vi "mass.vi"(1 "mass":dbl=1.0) -> (0 "urdf":string="<material>\n  <ambient> 0.705882 0.247059 0.000000 1.000000</ambient>\n</material>\n")   [LabVIEW 2012]
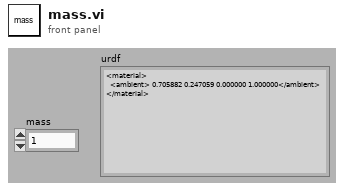
[diagram p1: front panel]
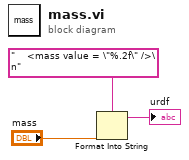
[diagram p0: block diagram]
diagram:
  n1 = Format Into String(format string="    <mass value = \"%.2f\" />\n", "mass") -> (resulting string=→"urdf":string)  [unwired: 2 in, 1 out]
